vi "MSEncoder Case-8-Wait.vi"(8 "error in (no error)":errorcluster, 9 "ParamValIn":variant, 11 "MSEncoder in":refnum<class "MSEncoder.lvclass">) -> (0 "error out":errorcluster, 3 "MSEncoder out":refnum<class "MSEncoder.lvclass">)   [LabVIEW 2018, in "MSEncoder.lvclass"]
uses:
  MSEncoder.lvclass
  Ctl/MSEditorParam wait.ctl
  MSEncoder.lvclass/MSEncoder.ctl
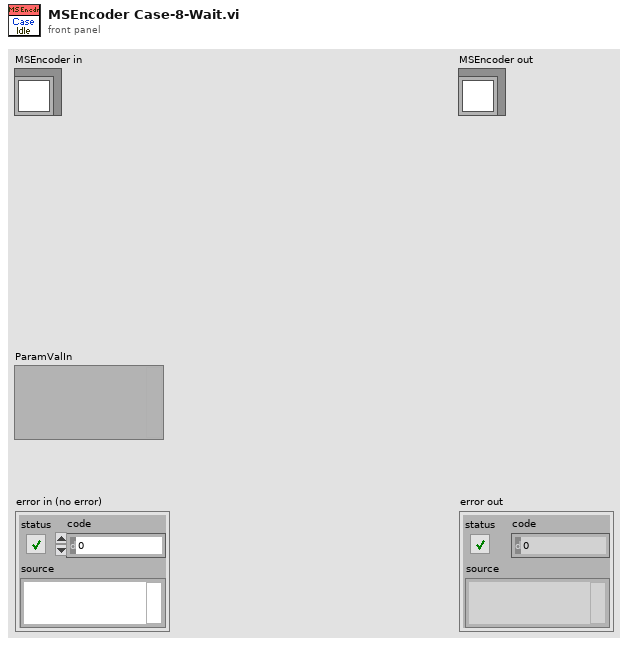
[diagram p1: front panel]
types:
  T1 = typedef "MSEditorParam wait.ctl" = cluster{"timeout":ext, "DI":u16, "edge":u16}
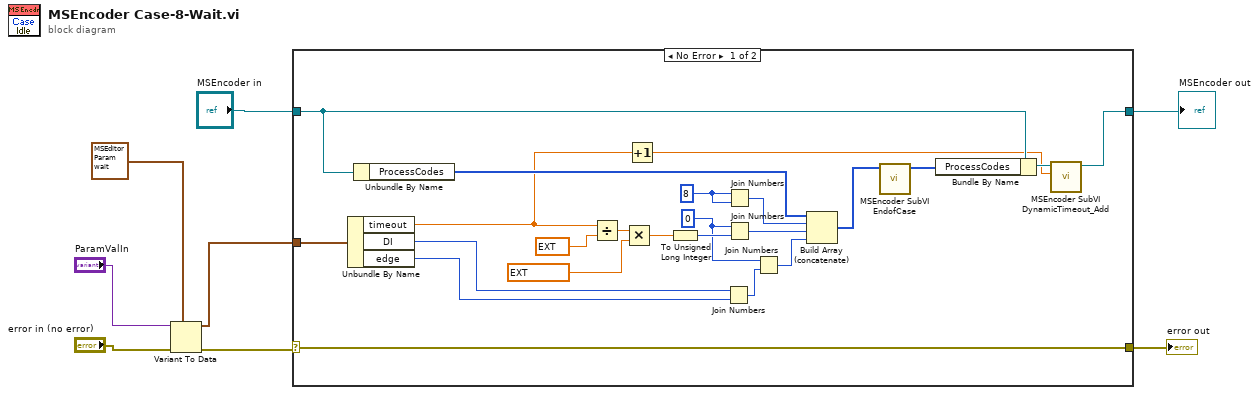
[diagram p0: block diagram]
diagram:
  n1 = Variant To Data(error in="error in (no error)", type=T1 {"timeout"=0.001, "DI"=0, "edge"=0} ("ParamValueType"), Variant="ParamValIn") -> (data=w3:T1, error out=w2:errorcluster)
  n2 = case shown="No Error" w2 {
    selector: w2 -> [w30 w33]
    tunnel: "MSEncoder in" -> [w29 w32]
    tunnel: [w30 w33] -> w8
    tunnel: [w16 w32] -> w6
    tunnel: w3 -> [w18 _]
    frame No Error {
      w11 = u32 0 ("hi")
      w27 = u32 8
      n3 = Unbundle By Name(w18) -> ("timeout"=w15:ext, "DI"=w13:u16, "edge"=w12:u16)
      n4 = Unbundle By Name(w29) -> ("ProcessCodes"=w31:u64[])
      n5 = Divide(x=w15, y=ext 1000.0) -> (x/y=w21:ext)
      n6 = Multiply(x=w21, y=ext 40000000.0) -> (x*y=w23:ext)
      n7 = Increment(x=w15) -> (x+1=w14:ext)
      n8 = To Unsigned Long Integer(number=w23) -> (unsigned 32bit integer=w22:u32)
      n9 = Join Numbers(hi=w13, lo=w12) -> ((hi.lo)=w10:u32)
      n10 = Join Numbers(hi=w27, lo=w27) -> ((hi.lo)=w26:u64)
      n11 = Join Numbers(hi=w11, lo=w22) -> ((hi.lo)=w25:u64)
      n12 = Join Numbers(hi=w11, lo=w10) -> ((hi.lo)=w9:u64)
      n13 = Build Array (concatenate)(w31, w26, w25, w9) -> (w19:u64[])
      n14 = call "MSEncoder SubVI EndofCase.vi"("Case codes"=w19) -> ("Case codes with end"=w28:u64[])  [unwired: 9 in, 1 out]
      n15 = Bundle By Name(cluster=w29, "ProcessCodes"=w28) -> (w17:refnum<class "MSEncoder.lvclass">)
      n16 = call "MSEncoder SubVI DynamicTimeout_Add.vi"("Timeout_ms"=w14, "MSEncoder"=w17) -> ("MSEncoder"=w16:refnum<class "MSEncoder.lvclass">)  [unwired: 8 in, 1 out]
    }
    frame Error {
    }
  }
  "error out" <- w8
  "MSEncoder out" <- w6
